vi "RestoreSetupLVSource.vi"   [LabVIEW 2020]
uses:
  <vilib>/Wiresmith Technology/G CLI/CLI Class/CLI.lvclass
  <userlib>/_OpenG.lib/file/file.llb/openg_file.lvlib
  <userlib>/_OpenG.lib/file/file.llb/Convert File Extension (Path)__ogtk.vi
  <userlib>/_OpenG.lib/lvzip/lvzip.llb/subVI/ZLIB Extract All Files To Dir (Path)__ogtk.vi
  <vilib>/Utility/config.llb/NI_LVConfig.lvlib
types:
  T1 = enum32{"Invalid", "Standard", "Closed", "Hidden", "Minimized", "Maximized"}
  T2 = typedef "NI_LVConfig.lvlib/Config Data RefNum.ctl" = refnum<k1>
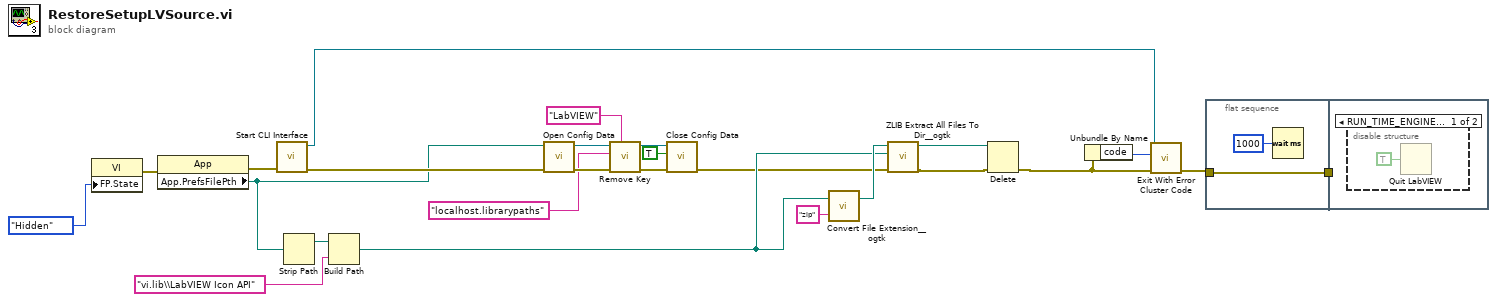
[diagram p0: block diagram]
diagram:
  n1 = property class="VI"("FP.State"=T1."Hidden" ("Front Panel Window:State")) -> (error out=w20:errorcluster)  [unwired: 2 in, 1 out]
  n2 = property class="App"(error in=w20) -> (error out=w19:errorcluster, "App.PrefsFilePth"=w4:path)  [unwired: 1 in, 1 out]
  n3 = call <vilib>:"Start CLI Interface.vi"("error in (no error)"=w19) -> ("error out"=w6:errorcluster, "CLI out"=w25:refnum<class "CLI.lvclass">)  [unwired: 7 in, 2 out]
  n4 = Strip Path(path=w4) -> (stripped path=w16:path)  [unwired: 1 out]
  n5 = Build Path(base path=w16, name or relative path="vi.lib\\LabVIEW Icon API" ("name")) -> (appended path=w14:path)
  n6 = call <vilib>:"Open Config Data.vi"("error in (no error)"=w6, "configuration file path"=w4) -> ("error out"=w10:errorcluster, "refnum"=w8:T2)  [unwired: 7 in, 1 out]
  n7 = call <vilib>:"Remove Key.vi"("section"="LabVIEW", "error in (no error)"=w10, "key"="localhost.librarypaths", "refnum"=w8) -> ("error out"=w9:errorcluster, "refnum out"=w7:T2)  [unwired: 5 in, 1 out]
  n8 = call <vilib>:"Close Config Data.vi"("error in (no error)"=w9, "write file if changed (T)"=TRUE, "refnum"=w7) -> ("error out"=w5:errorcluster)  [unwired: 7 in, 1 out]
  n9 = call-poly <userlib>:"Convert File Extension__ogtk.vi"("new ending (none)"="zip", "file name"=w14) -> ("new filename"=w15:path)  [unwired: 1 out]
  n10 = call-poly <userlib>:"ZLIB Extract All Files To Dir__ogtk.vi"("error in (no error)"=w5, "destination directory (archive name without ending)"=w14, "archive name (file dialog)"=w15) -> ("error out"=w13:errorcluster, "archive name out"=w11:path)  [unwired: 6 in, 1 out]
  n11 = Delete(path (use dialog)=w11, error in=w13) -> (error out=w12:errorcluster)  [unwired: 3 in, 2 out]
  n12 = Unbundle By Name(w12) -> ("code"=w22:i32)
  n13 = call <vilib>:"Exit With Error Cluster Code.vi"("error in (no error)"=w12, "No Error Code (0)"=w22, "CLI in"=w25) -> ("error out"=w23:errorcluster)  [unwired: 8 in]
  n14 = flat-sequence {
    tunnel: w23 -> [w27]
    tunnel: [w27] -> w24
    tunnel: w24 -> [_]
    frame #0 {
      n15 = Wait (ms)(milliseconds to wait=u32 1000) -> ()  [unwired: 1 out]
    }
    frame #1 {
      n16 = disable-structure shown="RUN_TIME_ENGINE==True" {
        frame condition #0 {
          n17 = Quit LabVIEW(quit? (T)=TRUE) -> ()
        }
        frame condition #1 (active) {
        }
      }
    }
  }
